vi "TDT-Write DO (method 2).vi"(0 "RPcox":refnum<k7>, 5 "Next Buffer":i32, 7 "Input array":bool[][](array[boolean]), 9 "Chans":i32[](array[numeric]), 11 "error in (no error)":errorcluster) -> (4 "RPcox (thru)":refnum<k7>, 15 "error out":errorcluster)   [LabVIEW 2020]
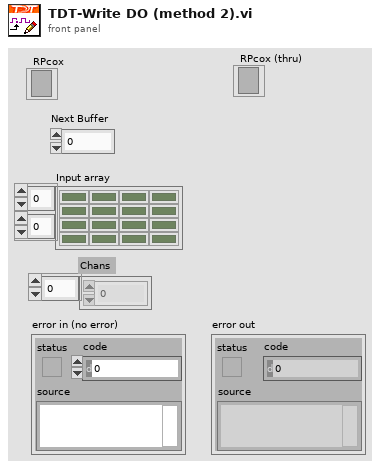
[diagram p1: front panel]
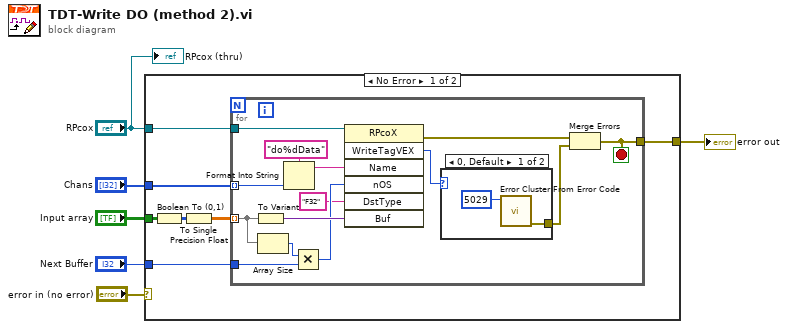
[diagram p0: block diagram]
diagram:
  n1 = case shown="No Error" "error in (no error)" {
    selector: "error in (no error)" -> [_ w30]
    tunnel: "Next Buffer" -> [w13 _]
    tunnel: "Input array" -> [w12 _]
    tunnel: "RPcox" -> [w11 _]
    tunnel: [w10 w30] -> w2
    tunnel: "Chans" -> [w9 _]
    frame No Error {
      n2 = Boolean To (0,1)(Boolean=w12) -> (0, 1=w8:i16[][])
      n3 = To Single Precision Float(number=w8) -> (single precision float=w7:sgl[][])
      n4 = for {
        tunnel: w11 -> [w27]
        tunnel: w7 -> [w18] mode=indexing
        tunnel: [w16] -> w10
        tunnel: w13 -> [w23]
        tunnel: w9 -> [w14] mode=indexing
        stop <- w16 stop-if-true
        n5 = To Variant(anything=w18) -> (Variant=w22:variant)
        n6 = Array Size(array=w18) -> (size(s)=w19:i32)
        n7 = Format Into String(format string="do%dData", w14) -> (resulting string=w25:string)  [unwired: 2 in, 1 out]
        n8 = Multiply(x=w19, y=w23) -> (x*y=w21:i32)
        n9 = invoke class="RPcoX" method="WriteTagVEX"(reference=w27, "Name"=w25, "nOS"=w21, "DstType"="F32", "Buf"=w22) -> (error out=w24:errorcluster, "WriteTagVEX"=w17:i32)  [unwired: 2 in, 5 out]
        n10 = case shown="0, Default" w17 {
          tunnel: [w28 _] -> w15
          frame 0, Default {
            n11 = call <vilib>:"Error Cluster From Error Code.vi"("error code (0)"=5029) -> ("error out"=w28:errorcluster)  [unwired: 8 in]
          }
          frame 1 {
          }
        }
        n12 = Merge Errors(w24, w15) -> (w16:errorcluster)
      }
    }
    frame Error {
    }
  }
  "error out" <- w2
  "RPcox (thru)" <- "RPcox"
